vi "rising edge.vi"(3 "Boolean input":bool) -> (1 "rising edge?":bool)   [LabVIEW 2021, in "RocketPlot.lvlib"]
uses:
  RocketPlot.lvlib
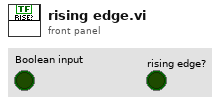
[diagram p1: front panel]
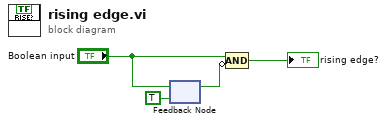
[diagram p0: block diagram]
diagram:
  n1 = feedback-in #1("Boolean input") -> ()
  n2 = feedback #1(TRUE ("Boolean input")) -> (w2:bool)
  n3 = Compound Arithmetic op=AND("Boolean input", invert w2) -> (→"rising edge?":bool)
